vi "Setup.vi"(8 "Error In":errorcluster, 11 "VI In":refnum<vi>) -> (0 "Error Out":errorcluster, 3 "VI Out":refnum<vi>)   [LabVIEW 2017, in "Tests.lvlib" / "Toolkit.lvlib"]
uses:
  Toolkit.lvlib
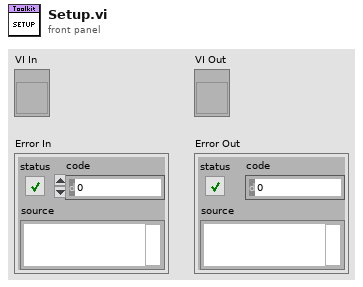
[diagram p1: front panel]
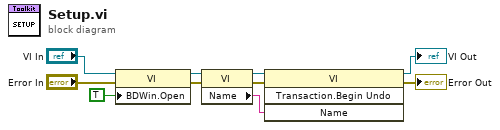
[diagram p0: block diagram]
diagram:
  n1 = property class="VI"(reference="VI In", error in="Error In", "BDWin.Open"=TRUE ("Block Diagram Window:Open")) -> (reference out=w7:refnum<vi>, error out=w3:errorcluster)
  n2 = property class="VI"(reference=w7, error in=w3) -> (reference out=w4:refnum<vi>, error out=w2:errorcluster, "Name"=w1:string)
  n3 = invoke class="VI" method="Transaction.Begin Undo"(reference=w4, error in=w2, "Name"=w1) -> (reference out=→"VI Out":refnum<vi>, error out=→"Error Out":errorcluster)  [unwired: 1 in, 2 out]
